vi "IncrementWrite.vi"(6 "Phidget ID":u64, 7 "Range (+-) (V)":dbl=60.0 min=1.0 max=60.0, 8 "error in (no error)":errorcluster, 9 "Ring":u16(ring) items=["Init", "Write"], 10 "Array":dbl[](array[numeric]), 11 "Keithley 2231 Name":refnum<visa-resource-name>) -> (0 "error in (no error) 2":errorcluster, 1 "WritingV":dbl, 2 "Voltage Back":dbl, 3 "Keithley 2231 Name Out":refnum<visa-resource-name>)   [LabVIEW 2019, in "2231A.lvclass"]
uses:
  2231A.lvclass
  <instrlib>/Phidgets/Phidget Digital Output/Phidget Digital Output.lvlib
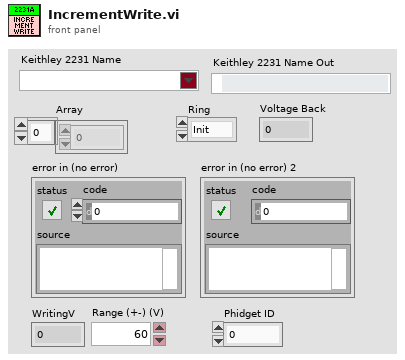
[diagram p1: front panel]
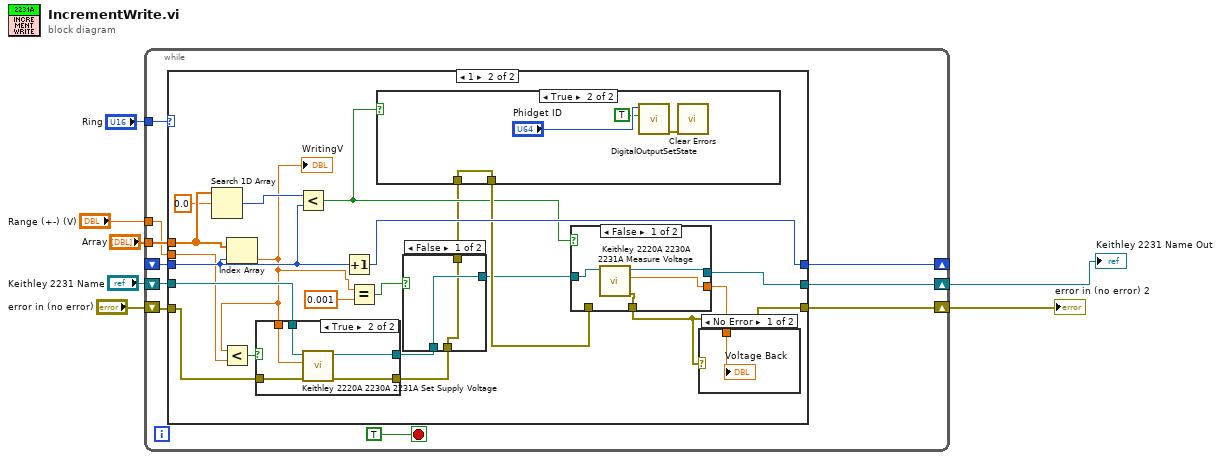
[diagram p0: block diagram]
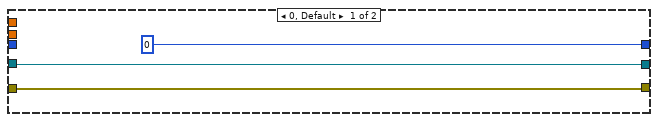
[diagram p2: hidden frame]
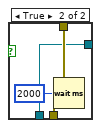
[diagram p3: hidden frame]
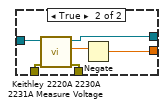
[diagram p7: hidden frame]
diagram:
  n1 = while {
    shift-right: [w16] -> w4
    shift-left: "error in (no error)" -> [w14]
    shift-right: [w17] -> w2
    shift-left: "Keithley 2231 Name" -> [w15]
    tunnel: "Array" -> [w13]
    tunnel: "Ring" -> [w12]
    shift-right: [w11] -> _
    shift-left: _ -> [w10]
    tunnel: "Range (+-) (V)" -> [w8]
    stop <- TRUE stop-if-true
    n2 = case shown="1" w12 {
      tunnel: [w19 w34] -> w17
      tunnel: [w18 w32] -> w16
      tunnel: w15 -> [w19 w41]
      tunnel: w14 -> [w18 w40]
      tunnel: w13 -> [_ w39]
      tunnel: [0 w33] -> w11
      tunnel: w10 -> [_ w36]
      tunnel: w8 -> [_ w30]
      frame 0, Default {
      }
      frame 1 {
        n3 = Search 1D Array(1D array=w39, element=0.0) -> (index of element=w37:i32)  [unwired: 1 in]
        n4 = Index Array(array=w39, index=w36) -> (element=w27:dbl)
        "WritingV" <- w27
        n5 = Less?(x=w27, y=w30) -> (x < y?=w31:bool)
        n6 = case shown="True" w31 {
          tunnel: w41 -> [w53 w58]
          tunnel: w40 -> [w52 w57]
          tunnel: w27 -> [_ w56]
          tunnel: [w53 w55] -> w24
          tunnel: [w52 w54] -> w23
          frame False {
          }
          frame True {
            n7 = call "Keithley 2220A 2230A 2231A Set Supply Voltage.vi"("error in (no error)"=w57, "Supply Voltage"=w56, "VISA resource name"=w58) -> ("error out"=w54:errorcluster, "VISA resource name out"=w55:refnum<visa-resource-name>)  [unwired: 7 in]
          }
        }
        n8 = Less?(x=w37, y=w36) -> (x < y?=w28:bool)
        n9 = Increment(x=w36) -> (x+1=w33:i32)
        n10 = Equal?(x=w27, y=0.001) -> (x = y?=w25:bool)
        n11 = case shown="False" w25 {
          tunnel: w24 -> [w43 w45]
          tunnel: w23 -> [w42 w46]
          tunnel: [w42 w46] -> w22
          tunnel: [w43 w45] -> w21
          frame False {
          }
          frame True {
            n12 = Wait (ms)(milliseconds to wait=u32 2000) -> ()  [unwired: 1 out]
          }
        }
        n13 = case shown="True" w28 {
          tunnel: w22 -> [w47 w48]
          tunnel: [w47 w48] -> w29
          frame False {
          }
          frame True {
            n14 = call <instrlib>:"DigitalOutputSetState.vi"("State"=TRUE, "Device In"="Phidget ID") -> ("error out"=w49:errorcluster)  [unwired: 7 in, 1 out]
            n15 = call <vilib>:"Clear Errors.vi"("error in (no error)"=w49) -> ()  [unwired: 5 in, 2 out]
          }
        }
        n16 = case shown="False" w28 {
          tunnel: [w61 w69] -> w35
          tunnel: w21 -> [w63 w68]
          tunnel: [w62 w66] -> w34
          tunnel: [w60 w65] -> w32
          tunnel: w29 -> [_ w64]
          frame False {
            n17 = call "Keithley 2220A 2230A 2231A Measure Voltage.vi"("VISA resource name"=w63) -> ("error out"=w60:errorcluster, "Measured Voltage"=w61:sgl, "VISA resource name out"=w62:refnum<visa-resource-name>)  [unwired: 8 in]
          }
          frame True {
            n18 = call "Keithley 2220A 2230A 2231A Measure Voltage.vi"("error in (no error)"=w64, "VISA resource name"=w68) -> ("error out"=w65:errorcluster, "Measured Voltage"=w67:sgl, "VISA resource name out"=w66:refnum<visa-resource-name>)  [unwired: 7 in]
            n19 = Negate(x=w67) -> (-x=w69:sgl)
          }
        }
        n20 = case shown="No Error" w32 {
          tunnel: w35 -> [w59 _]
          frame No Error {
            "Voltage Back" <- w59
          }
          frame Error {
          }
        }
      }
    }
  }
  "error in (no error) 2" <- w4
  "Keithley 2231 Name Out" <- w2
